vi "Freq-Mod_Host.vi"() -> ()   [LabVIEW 2012]
uses:
  <vilib>/FPGAPlugInAG/PCI-7831R/niLvFpga_Open_PCI-7831R.vi
  <vilib>/rvi/errors/niLvFpgaMergeErrorWithErrorCode.vi
  <vilib>/rvi/errors/niLvFpgaAdjustHostInterfaceError.vi
  <vilib>/Utility/error.llb/Error Cluster From Error Code.vi
  <vilib>/FPGAPlugInAG/PCI-7831R/niLvFpga_Abort_PCI-7831R.vi
  <vilib>/FPGAPlugInAG/PCI-7831R/niLvFpga_Close_PCI-7831R.vi
  <vilib>/rvi/interface/nirviOpenFPGA/nirviOpenFPGA.xnode
  SB130-XPS/Documents/FPGA-project-apporach-retraction/FPGA Bitfiles/Apporach-Retract_FPGATarget2_Freq-ModPrototyp_TlfskMu8vfU.lvbitx
  Freq-Mod_Prototype.vi
  <vilib>/rvi/interface/nirviReadWriteControl/nirviReadWriteControl.xnode
  <vilib>/rvi/interface/nirviMethod/nirviMethod.xnode
  <vilib>/rvi/interface/nirviCloseFPGA/nirviCloseFPGA.xnode
  NiFpgaLv.dll
panel:
  out "R (Amplitude) 1":dbl(graph)
  out "Frequency 1":dbl(graph)
  in  "stop":bool
  in  "K Constant":fxp<+/-,64,32>
  in  "Time Constant [s]":dbl=2.5 min=0.0 step=0.0001 format="%.2f"
  in  "Filter Rolloff":enum16{"20 dB", "40 dB", "60 dB", "80 dB"}(ring)
  in  "Sampling Frequency":i32=200000
  in  "Lock In PLL\nNominal Frequency":i32=30000
  out "VCO Output":dbl(graph)
  in  "Stages":i32=1
  in  "Decimation":i32=586
  in  "Dec2":i32=256
  in  "Dec1":i32=1
  out "R (Amplitude)":dbl(graph)
  out "Frequency":dbl(graph)
  out "Degrees":dbl
  in  "Phase Setpoint":fxp<+/-,64,32>=1.5708000001031905
  in  "alpha [U16.-2]":fxp<+/-,64,26>=0.00999999999839929
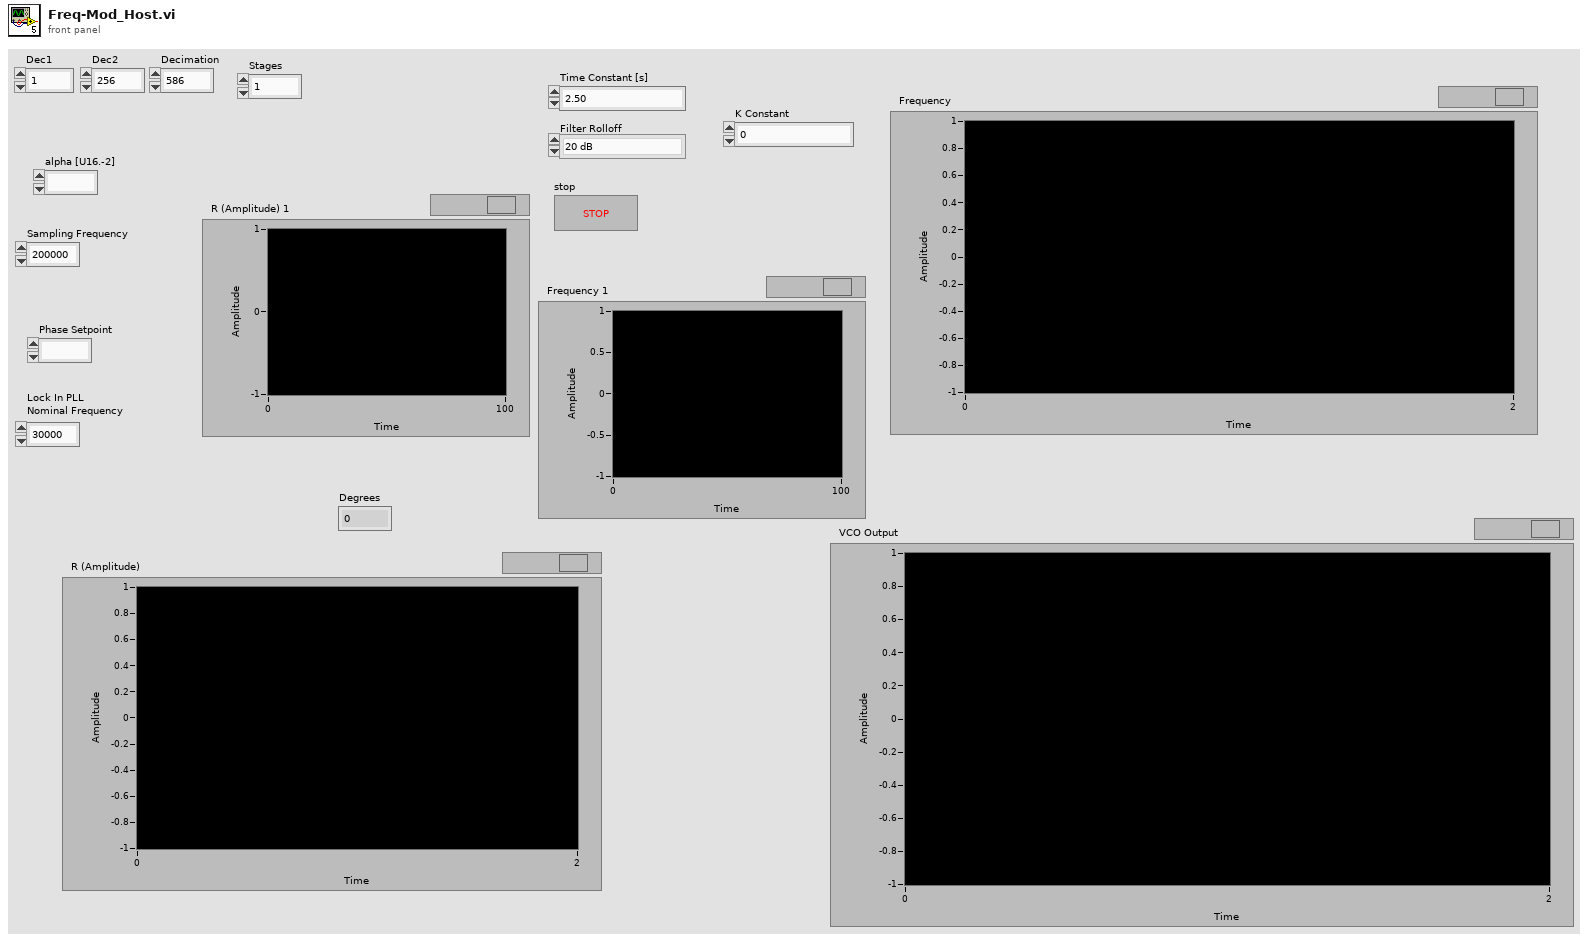
[diagram p1: front panel]
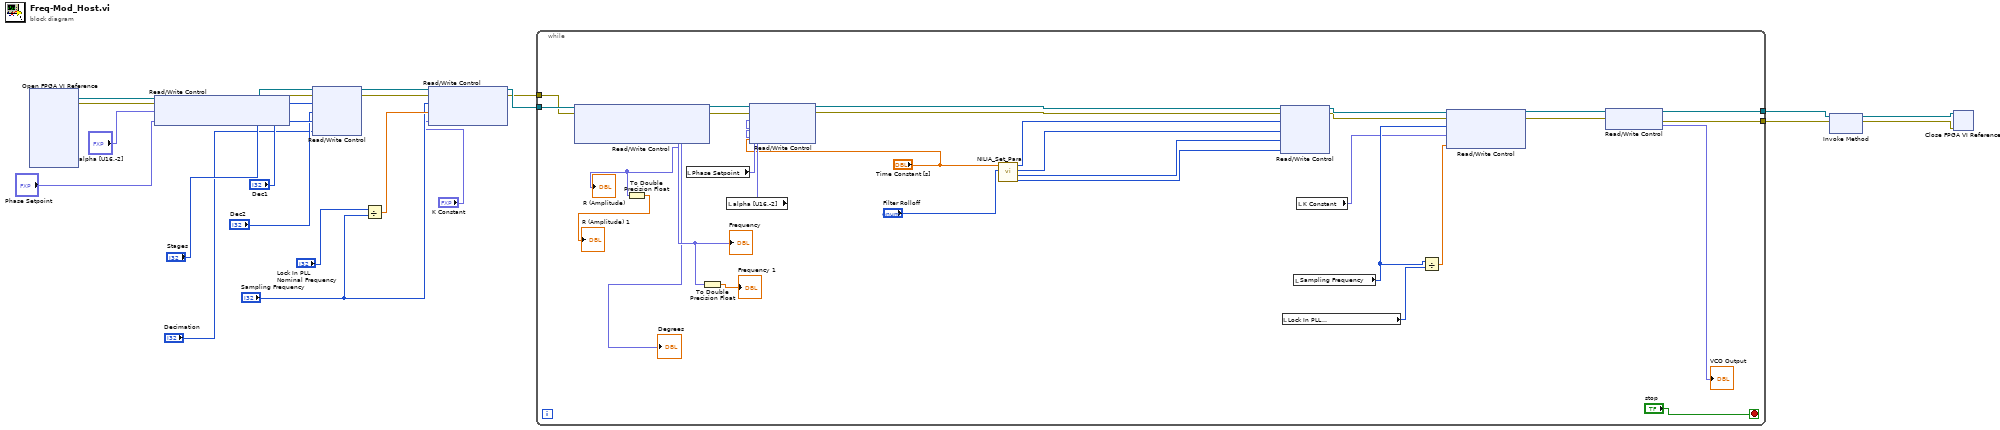
[diagram p0: block diagram]
diagram:
  n1 = xnode "Open FPGA VI Reference"() -> ("FPGA VI Reference Out"=w22:refnum<k20>, "error out"=w21:errorcluster)  [unwired: 2 in]
  n2 = xnode "Read/Write Control"("FPGA VI Reference In"=w22, "error in"=w21, "alpha [U16.-2] 2"="alpha [U16.-2]", "phase setpoint 2"="Phase Setpoint") -> ("FPGA VI Reference Out"=w14:refnum<k20>, "error out"=w13:errorcluster)
  n3 = xnode "Read/Write Control"("FPGA VI Reference In"=w14, "error in"=w13, "dec1"="Dec1", "dec2"="Dec2", "stages"="Stages", "decimation"="Decimation") -> ("FPGA VI Reference Out"=w11:refnum<k20>, "error out"=w12:errorcluster)
  n4 = Divide(x="Lock In PLL\nNominal Frequency", y="Sampling Frequency") -> (x/y=w10:dbl)
  n5 = xnode "Read/Write Control"("FPGA VI Reference In"=w11, "error in"=w12, "Sampling Frequency"="Sampling Frequency", "Nominal Freq LIA"=w10, "K Constant"="K Constant") -> ("FPGA VI Reference Out"=w7:refnum<k20>, "error out"=w6:errorcluster)
  n6 = while {
    tunnel: w7 -> [w50]
    tunnel: w6 -> [w49]
    tunnel: [w45] -> w3
    tunnel: [w44] -> w2
    stop <- "stop" stop-if-true
    n7 = xnode "Read/Write Control"("FPGA VI Reference In"=w50, "error in"=w49) -> ("FPGA VI Reference Out"=w43:refnum<k20>, "error out"=w42:errorcluster, "Degrees"=→"Degrees":fxp<+,4,1>, "F Graph"=w26:fxp<+,14,17>, "R (Amplitude)"=w23:fxp<+,7,1>)
    "Frequency" <- w26
    "R (Amplitude)" <- w23
    n8 = To Double Precision Float(number=w23) -> (double precision float=→"R (Amplitude) 1":dbl)
    n9 = local read "Phase Setpoint"() -> (w30:fxp<+/-,64,32>)
    n10 = To Double Precision Float(number=w26) -> (double precision float=→"Frequency 1":dbl)
    n11 = local read "alpha [U16.-2]"() -> (w39:fxp<+/-,64,26>)
    n12 = xnode "Read/Write Control"("FPGA VI Reference In"=w43, "error in"=w42, "alpha [U16.-2] 2"=w39, "phase setpoint 2"=w30, "Time Constant"="Time Constant [s]") -> ("FPGA VI Reference Out"=w41:refnum<k20>, "error out"=w40:errorcluster)
    n13 = call "NILIA_Set_Para.vi"("rolloff"="Filter Rolloff", "TC [sec]"="Time Constant [s]") -> ("3rd stages"=w32:i32, "3rd decimation"=w33:i32, "2nd decimation"=w34:i32, "1st decimation"=w35:i32)  [unwired: 5 in, 1 out]
    n14 = xnode "Read/Write Control"("FPGA VI Reference In"=w41, "error in"=w40, "dec1"=w35, "dec2"=w34, "stages"=w33, "decimation"=w32) -> ("FPGA VI Reference Out"=w38:refnum<k20>, "error out"=w37:errorcluster)
    n15 = local read "Lock In PLL\nNominal Frequency"() -> (w47:i32)
    n16 = local read "Sampling Frequency"() -> (w48:i32)
    n17 = local read "K Constant"() -> (w31:fxp<+/-,64,32>)
    n18 = Divide(x=w48, y=w47) -> (x/y=w46:dbl)
    n19 = xnode "Read/Write Control"("FPGA VI Reference In"=w38, "error in"=w37, "Sampling Frequency"=w48, "K Constant"=w31, "Nominal Freq LIA"=w46) -> ("FPGA VI Reference Out"=w53:refnum<k20>, "error out"=w52:errorcluster)
    n20 = xnode "Read/Write Control"("FPGA VI Reference In"=w53, "error in"=w52) -> ("FPGA VI Reference Out"=w45:refnum<k20>, "error out"=w44:errorcluster, "sin(z) [I16.2] 2"=→"VCO Output":fxp<+/-,10,1>)
  }
  n21 = xnode "Invoke Method"("FPGA VI Reference In"=w3, "error in"=w2) -> ("FPGA VI Reference Out"=w5:refnum<k20>, "error out"=w4:errorcluster)
  n22 = xnode "Close FPGA VI Reference"("FPGA VI Reference In"=w5, "error in"=w4) -> ()  [unwired: 1 out]
